vi "CuboMagico.vi"() -> ()   [LabVIEW 2020]
panel:
  out "Suma":i32
  out "Cuadrado":i32[][](array[numeric])
  out "Boolean":bool
  in  "Numero":string(combo)
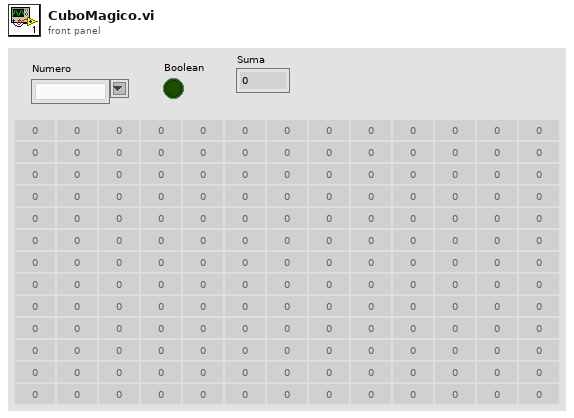
[diagram p1: front panel]
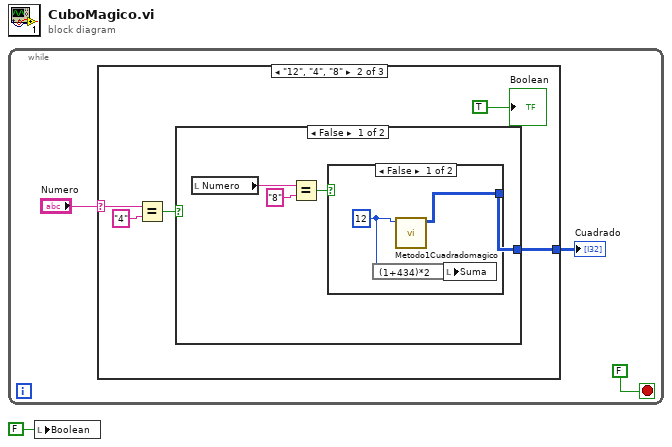
[diagram p0: block diagram]
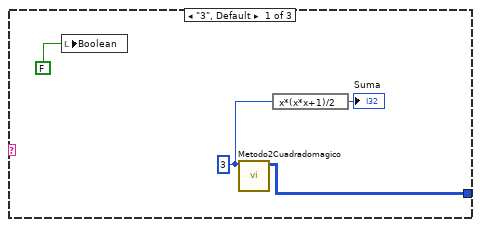
[diagram p2: hidden frame]
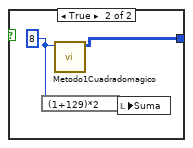
[diagram p3: hidden frame]
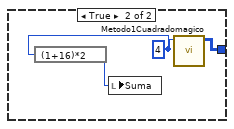
[diagram p4: hidden frame]
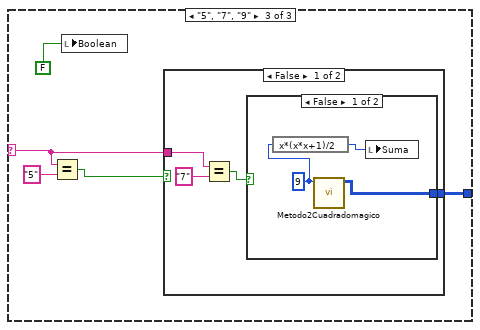
[diagram p5: hidden frame]
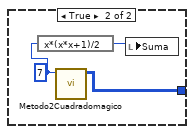
[diagram p6: hidden frame]
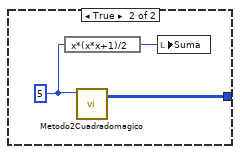
[diagram p7: hidden frame]
diagram:
  n1 = while {
    stop <- FALSE stop-if-true
    n2 = case shown="\"12\", \"4\", \"8\"" "Numero" {
      selector: "Numero" -> [_ w12 w27]
      tunnel: [w7 w9 w28] -> w2
      frame "3", Default {
        w5 = 3 ("Numero")
        n3 = local write "Boolean"(FALSE) -> ()
        n4 = call "Metodo2Cuadradomagico.vi"("NumeroImpar"=w5) -> ("Array"=w7:i32[][])  [unwired: 10 in]
        n5 = expression code="x*(x*x+1)/2"(w5) -> (→"Suma":i32)
      }
      frame "12", "4", "8" {
        n6 = Equal?(x=w12, y="4") -> (x = y?=w10:bool)
        n7 = case shown="False" w10 {
          tunnel: [w14 w26] -> w9
          frame False {
            n8 = local read "Numero"() -> (w17:string)
            n9 = Equal?(x=w17, y="8") -> (x = y?=w15:bool)
            n10 = case shown="False" w15 {
              tunnel: [w20 w23] -> w14
              frame False {
                w19 = 12 ("N 2")
                n11 = expression code="(1+434)*2"(w19) -> (w18:i32)
                n12 = call "Metodo1Cuadradomagico.vi"("NumeroN4"=w19) -> ("Array 2"=w20:i32[][])  [unwired: 10 in]
                n13 = local write "Suma"(w18) -> ()
              }
              frame True {
                w22 = 8 ("N 2")
                n14 = expression code="(1+129)*2"(w22) -> (w21:i32)
                n15 = call "Metodo1Cuadradomagico.vi"("NumeroN4"=w22) -> ("Array 2"=w23:i32[][])  [unwired: 10 in]
                n16 = local write "Suma"(w21) -> ()
              }
            }
          }
          frame True {
            w25 = 4 ("N 2")
            n17 = expression code="(1+16)*2"(w25) -> (w24:i32)
            n18 = local write "Suma"(w24) -> ()
            n19 = call "Metodo1Cuadradomagico.vi"("NumeroN4"=w25) -> ("Array 2"=w26:i32[][])  [unwired: 10 in]
          }
        }
        "Boolean" <- TRUE
      }
      frame "5", "7", "9" {
        n20 = Equal?(x=w27, y="5") -> (x = y?=w30:bool)
        n21 = local write "Boolean"(FALSE) -> ()
        n22 = case shown="False" w30 {
          tunnel: [w32 w44] -> w28
          tunnel: w27 -> [w35 _]
          frame False {
            n23 = Equal?(x=w35, y="7") -> (x = y?=w33:bool)
            n24 = case shown="False" w33 {
              tunnel: [w38 w41] -> w32
              frame False {
                w36 = 9 ("Numero")
                n25 = expression code="x*(x*x+1)/2"(w36) -> (w37:i32)
                n26 = call "Metodo2Cuadradomagico.vi"("NumeroImpar"=w36) -> ("Array"=w38:i32[][])  [unwired: 10 in]
                n27 = local write "Suma"(w37) -> ()
              }
              frame True {
                w40 = 7 ("Numero")
                n28 = expression code="x*(x*x+1)/2"(w40) -> (w39:i32)
                n29 = call "Metodo2Cuadradomagico.vi"("NumeroImpar"=w40) -> ("Array"=w41:i32[][])  [unwired: 10 in]
                n30 = local write "Suma"(w39) -> ()
              }
            }
          }
          frame True {
            w42 = 5 ("Numero")
            n31 = expression code="x*(x*x+1)/2"(w42) -> (w43:i32)
            n32 = call "Metodo2Cuadradomagico.vi"("NumeroImpar"=w42) -> ("Array"=w44:i32[][])  [unwired: 10 in]
            n33 = local write "Suma"(w43) -> ()
          }
        }
      }
    }
    "Cuadrado" <- w2
  }
  n34 = local write "Boolean"(FALSE) -> ()
